vi "test Copy To Larger Destinationvi.vi"(8 "error in (no error)":errorcluster, 11 "TestCase in":refnum<class "Data Manipulation Tests.lvclass">) -> (0 "error out":errorcluster, 3 "TestCase out":refnum<class "Data Manipulation Tests.lvclass">)   [LabVIEW 2017, in "Pointer Tests.lvlib" / "Data Manipulation Tests.lvclass"]
uses:
  Data Manipulation Tests.lvclass
  Source/Classes/Pointer/Pointer.lvclass/Pointer.ctl
  Source/Classes/Pointer/Public/New/New (4B).vi
  Source/Classes/Pointer/Public/Write/Write (1D I32).vi
  Source/Classes/Pointer/Public/New/New (8B).vi
  Source/Classes/Pointer/Public/Read/Read (1D I32).vi
  Source/Classes/Pointer/Private/Allocate.vi
  Source/Classes/Pointer/Public/Write (No Check)/Write (No Check 1D I32).vi
  Source/Classes/Pointer/Protected/Parameter Checking/Check Null Pointer.vi
  Source/Classes/Pointer/Protected/Parameter Checking/Check Subset (Power of 2).vi
  Source/Classes/Pointer/API/Accessors/Get Size.vi
  Source/Classes/Pointer/API/Copy Pointer Data.vi
  Source/Classes/Pointer/Public/Read (No Check)/Read (No Check 1D I32).vi
  Source/Classes/Pointer/Private/Deallocate.vi
  Source/Classes/Pointer/API/Accessors/Set Address.vi
  Source/Classes/Pointer/API/Accessors/Set Size.vi
  Source/Classes/Pointer/Private/Set Internal.vi
  Source/Classes/Pointer/API/Accessors/Get Address.vi
  Source/Classes/Pointer/Protected/Errors.vi
  Source/Classes/Pointer/Protected/Error VIs/Null Pointer.vi
  Source/Classes/Pointer/Protected/Error VIs/Out of Bounds.vi
  Source/Classes/Pointer/Private/Count to Size.vi
  Source/Classes/Pointer/Public/Copy (No Check).vi
  Source/Classes/Pointer/Protected/Parameter Checking/Check Subset.vi
  Source/Classes/Pointer/Protected/Get Internal.vi
  Source/Classes/Pointer/Protected/Error VIs/Zone.vi
  Source/Classes/Pointer/Protected/Error Building/Create Error.vi
  Source/VIs/Write String into Source.vi
  Source/Classes/Pointer/Protected/Error Building/Write Pointer Size.vi
  Source/VIs/Write Number into Source.vi
  Source/VIs/VIs for Poly/Write U64 into Source.vi
  Source/Constants/Constants.vi
  Source/Constants/Library Name.vi
  Source/Classes/Pointer/Protected/Error Building/Get Error Info.vi
  Source/VIs/Create Error Cluster.vi
  Source/VIs/VIs for Poly/Create Error Cluster (256B).vi
  Source/VIs/Set Error Status.vi
  Source/VIs/Set Error Code.vi
  Source/VIs/Set Error Source.vi
  Source/Classes/Pointer/Pointer.lvclass
  <vilib>/addons/_JKI Toolkits/VI Tester/TestCase.llb/TestCase.lvclass
  C:/Program Files (x86)/National Instruments/LabVIEW 2017/vi.lib/addons/_JKI Toolkits/VI Tester/TestCase.llb/TestCase.lvclass
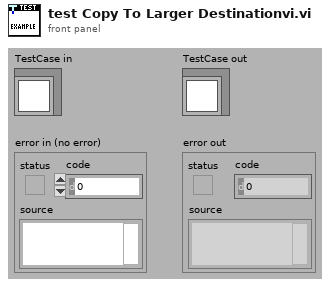
[diagram p1: front panel]
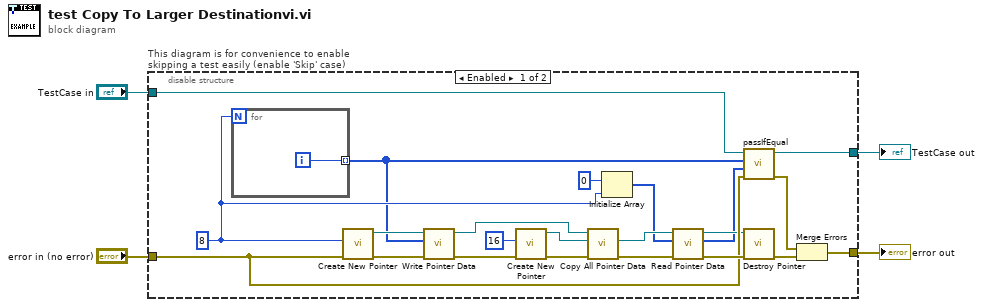
[diagram p0: block diagram]
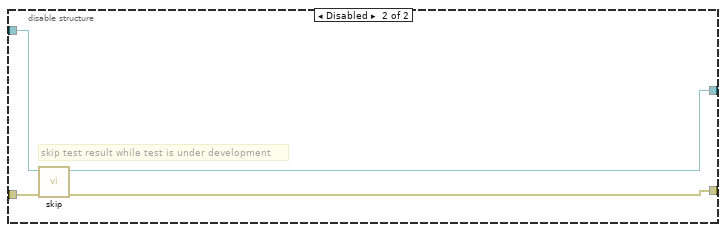
[diagram p2: hidden frame]
diagram:
  n1 = disable-structure "This diagram is for convenience to enable skipping a test easily (enable 'Skip' case)" shown="Enabled" {
    disable-tunnel: "TestCase in" -> [w17 w31]
    disable-tunnel: [w16 w29] -> w1
    disable-tunnel: [w20 w30] -> w3
    disable-tunnel: "error in (no error)" -> [w9 w28]
    frame Enabled {
      w15 = u64 8 ("count (1)")
      n2 = for {
        N: w15 -> [_]
        tunnel: [w27] -> w5 mode=indexing
        i -> [w27]
      }
      n3 = call-poly "Create New Pointer.vi"("error in (no error)"=w9, "count (1)"=w15) -> ("error out"=w23:errorcluster, "Pointer"=w26:refnum<class "Pointer.lvclass">)  [unwired: 8 in]
      n4 = call-poly "Write Pointer Data.vi"("error in (no error)"=w23, "buffer in"=w5, "Pointer in"=w26) -> ("error out"=w22:errorcluster, "Pointer out"=w25:refnum<class "Pointer.lvclass">)  [unwired: 5 in, 2 out]
      n5 = call-poly "Create New Pointer.vi"("error in (no error)"=w22, "count (1)"=u64 16) -> ("error out"=w21:errorcluster, "Pointer"=w24:refnum<class "Pointer.lvclass">)  [unwired: 8 in]
      n6 = call "Copy All Pointer Data.vi"("error in (no error)"=w21, "dst Pointer in"=w24, "src Pointer in"=w25) -> ("error out"=w12:errorcluster, "dst Pointer out"=w18:refnum<class "Pointer.lvclass">)  [unwired: 6 in, 1 out]
      n7 = Initialize Array(0 ("element"), w15) -> (w13:i32[])
      n8 = call-poly "Read Pointer Data.vi"("error in (no error)"=w12, "buffer in"=w13, "Pointer in"=w18) -> ("error out"=w11:errorcluster, "buffer out"=w6:i32[], "Pointer out"=w7:refnum<class "Pointer.lvclass">)  [unwired: 5 in, 1 out]
      n9 = call-dynamic "passIfEqual.vi"("error in (no error)"=w9, "y"=w6, "x"=w5, "TestCase in"=w17) -> ("error out"=w10:errorcluster, "TestCase out"=w16:refnum<class "Data Manipulation Tests.lvclass">)  [unwired: 6 in]
      n10 = call "Destroy Pointer.vi"("error in (no error)"=w11, "Pointer in"=w7) -> ("error out"=w8:errorcluster)  [unwired: 8 in, 1 out]
      n11 = Merge Errors(w10, w8) -> (w20:errorcluster)
    }
    frame Disabled {
      # "skip test result while test is under development"
      n12 = call <vilib>:"skip.vi"("error in (no error)"=w28, "TestCase in"=w31) -> ("error out"=w30:errorcluster, "TestCase out"=w29:refnum<class "Data Manipulation Tests.lvclass">)  [unwired: 8 in]
    }
  }
  "error out" <- w3
  "TestCase out" <- w1
